vi "Target_9.vi"   [LabVIEW 2020]
uses:
  <vilib>/Platform/TimedLoop/XDataNode/timing_clust.ctl
  <vilib>/Platform/TimedLoop/XDataNode/nitl_modes.ctl
  <vilib>/Platform/TimedLoop/XDataNode/wakeup.ctl
  <vilib>/platform/TimedLoop/XDataNode/XDataNode.xnode
  <vilib>/Platform/TimedLoop/XDataNode/XDNodeRunTimeDep.lvlib
types:
  T1 = typedef "XDNodeRunTimeDep.lvlib/timing_clust.ctl" = cluster{"Expected End [f-1]":u64, "Actual End [f-1]":u64, "Finished Late? [f-1]":bool, "Expected End [i-1]":u64, "Actual End [i-1]":u64, "Finished Late? [i-1]":bool, "Expected Start [i]":u64, "Actual Start [i]":u64, "Expected Start [f]":u64, "Actual Start [f]":u64, "Source Name":string, "Structure Name":string, "Period":i64, "Deadline":i64, "Offset":i64, "Start":i64, "Priority":i32, "Timeout":i32, "Mode":T2, "Wakeup Reason":T3, "Error":errorcluster, "Source Type":string, "Secondary Source Type":string, "Global End Time":u64, "Global Start Time":u64, "Frame Duration":u64, "Iteration Duration":u64, "Assigned CPU":i32, "I/O Scan Engine Mode":u32}
  T2 = typedef "XDNodeRunTimeDep.lvlib/nitl_modes.ctl" = enum32{"No Change", "Process missed periods, maintain original phase", "Discard missed periods, maintain original phase", "Process missed periods, ignore original phase", "Discard missed periods, ignore original phase"}
  T3 = typedef "XDNodeRunTimeDep.lvlib/wakeup.ctl" = enum32{"Normal", "Aborted", "Asynchronous wakeup", "Timing source error", "Timed loop error", "Timeout"}
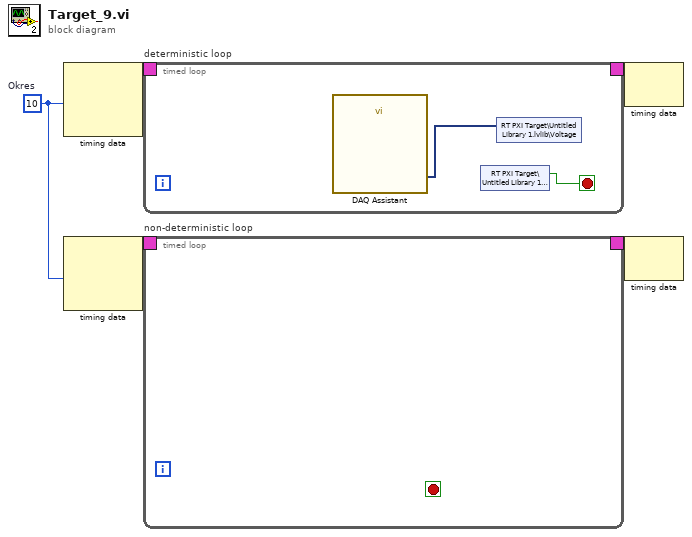
[diagram p0: block diagram]
diagram:
  w1 = i64 10  # Okres
  n1 = node-c288 ("Input Node")(w1) -> (w5:T1)  [unwired: 2 in]
  n2 = node-c288 ("Input Node")(w1) -> (w3:T1)  [unwired: 2 in]
  n3 = timed-loop "deterministic loop" {
    timing: w5 -> [_]
    timing-out: [_] -> w4
    stop <- w6 stop-if-true
    n4 = call "DAQ Assistant"() -> ("data"=w7:dynamicdata)  [unwired: 17 in, 2 out]
    n5 = shared-variable "RT PXI Target\\Untitled Library 1.lvlib\\Stop"() -> (w6:bool)  [unwired: 1 in, 1 out]
    n6 = shared-variable "RT PXI Target\\Untitled Library 1.lvlib\\Voltage"(w7) -> ()  [unwired: 1 in, 1 out]
  }
  n7 = timed-loop "non-deterministic loop" {
    timing: w3 -> [_]
    timing-out: [_] -> w2
    stop <- _ stop-if-true
  }
  n8 = node-c288 ("Output Node")(w4) -> ()  [unwired: 1 out]
  n9 = node-c288 ("Output Node")(w2) -> ()  [unwired: 1 out]
